vi "writeToXML.vi"(8 "error in (no error)":errorcluster, 10 "Class Label":string="Zenith", 11 "Zenith in":refnum<class "Zenith.lvclass">) -> (0 "error out":errorcluster, 2 "XML out":string="<Zenith>\n  <currentZD_deg>0</currentZD_deg>\n  <elZenithLimit_deg>0</elZenithLimit_deg>\n  <inBlindSpotIsTrue>false</inBlindSpotIsTrue>\n  <timeToBlindSpot_min>0</timeToBlindSpot_min>\n  <timeToBlindSpotExit_min>0</timeToBlindSpotExit_min>\n</Zenith>", 3 "Zenith out":refnum<class "Zenith.lvclass">)   [LabVIEW 2022 SP3, in "TCSDataDefinitions.lvlib" / "TCSPublicStatus.lvlib" / "Limits.lvlib" / "Zenith.lvclass"]
uses:
  Zenith.lvclass
  <userlib>/Common/UnitsAndXML/FlattenItemWithUnitToXML/FlattenPlaneAngleToXML/PlaneAngleUnit.ctl
  <userlib>/Common/UnitsAndXML/FlattenItemWithUnitToXML/FlattenTimeToXML/TimeUnit.ctl
  Zenith.lvclass/Zenith.ctl
  <userlib>/Common/UnitsAndXML/UnitsAndXML.lvlib
  <userlib>/Common/XML/XMLGenerator/XMLGenerator.lvclass
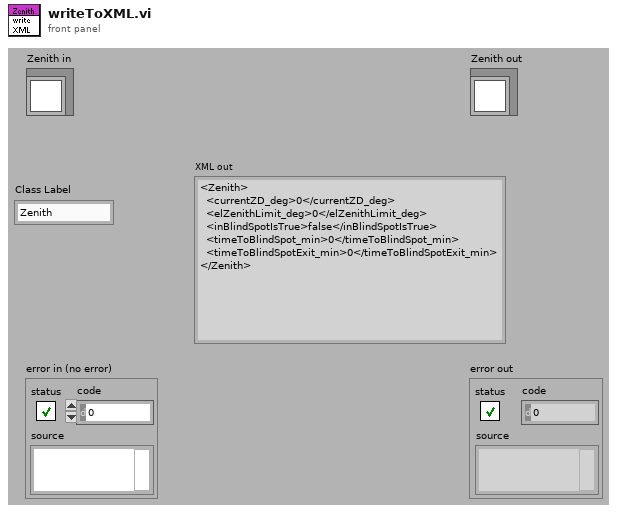
[diagram p1: front panel]
types:
  T1 = typedef "UnitsAndXML.lvlib/TimeUnit.ctl" = enum16{"s", "d", "h", "min", "a"}
  T2 = typedef "UnitsAndXML.lvlib/PlaneAngleUnit.ctl" = enum16{"rad", "deg", "'", "\""}
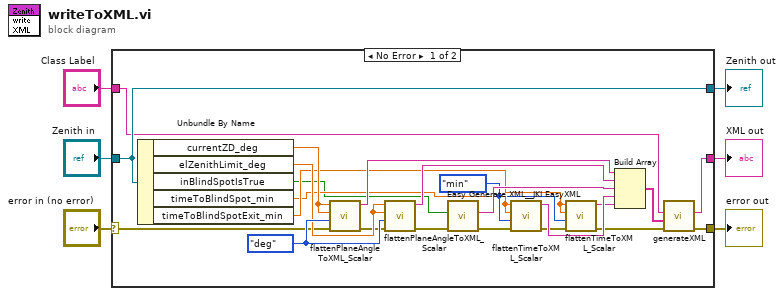
[diagram p0: block diagram]
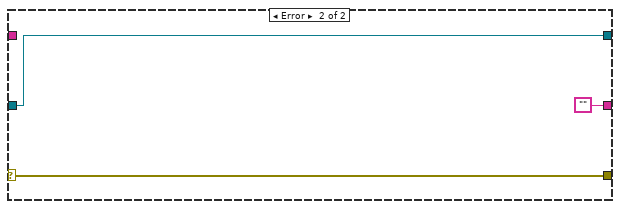
[diagram p2: hidden frame]
diagram:
  n1 = case shown="No Error" "error in (no error)" {
    selector: "error in (no error)" -> [w24 w32]
    tunnel: [w10 w32] -> w5
    tunnel: [w29 w31] -> w3
    tunnel: "Zenith in" -> [w29 w31]
    tunnel: "Class Label" -> [w8 _]
    tunnel: [w7 ""] -> w1
    frame No Error {
      w16 = TimeUnit."min" ("timeUnitInXML")
      w27 = PlaneAngleUnit."deg" ("planeAngleUnitInXML")
      n2 = Unbundle By Name(w29) -> ("currentZD_deg"=w28:dbl[unit], "elZenithLimit_deg"=w26:dbl[unit], "inBlindSpotIsTrue"=w12:bool, "timeToBlindSpot_min"=w17:dbl[unit], "timeToBlindSpotExit_min"=w18:dbl[unit])
      n3 = call <userlib>:"flattenPlaneAngleToXML_Scalar.vi"("error in (no error)"=w24, "planeAngleUnitInXML"=w27, "planeAngleAgain"=w28, "planeAngle"=w28) -> ("error out"=w25:errorcluster, "xmlString"=w23:string)  [unwired: 6 in]
      n4 = call <userlib>:"flattenPlaneAngleToXML_Scalar.vi"("error in (no error)"=w25, "planeAngleUnitInXML"=w27, "planeAngleAgain"=w26, "planeAngle"=w26) -> ("error out"=w13:errorcluster, "xmlString"=w22:string)  [unwired: 6 in]
      n5 = call <vilib>:"Easy Generate XML__JKI EasyXML.vi"("error in (no error)"=w13, "LabVIEW Data"=w12) -> ("error out"=w14:errorcluster, "XML String"=w21:string)  [unwired: 8 in]
      n6 = call <userlib>:"flattenTimeToXML_Scalar.vi"("error in (no error)"=w14, "timeUnitInXML"=w16, "timeAgain"=w17, "time"=w17) -> ("error out"=w15:errorcluster, "xmlString"=w20:string)  [unwired: 6 in]
      n7 = call <userlib>:"flattenTimeToXML_Scalar.vi"("error in (no error)"=w15, "timeUnitInXML"=w16, "timeAgain"=w18, "time"=w18) -> ("error out"=w11:errorcluster, "xmlString"=w19:string)  [unwired: 6 in]
      n8 = Build Array(w23, w22, w21, w20, w19) -> (w9:string[])
      n9 = call <userlib>:"generateXML.vi"("error in"=w11, "childrenXML"=w9, "elementName"=w8) -> ("error out"=w10:errorcluster, "XML out"=w7:string)  [unwired: 6 in, 1 out]
    }
    frame Error {
    }
  }
  "error out" <- w5
  "Zenith out" <- w3
  "XML out" <- w1
